vi "tagbit.vi"(9 "tag":string="A_B_C_D") -> (3 "tag cell":string[](array[string]))   [LabVIEW 2011]
uses:
  <vilib>/regexp/Match Regular Expression.xnode
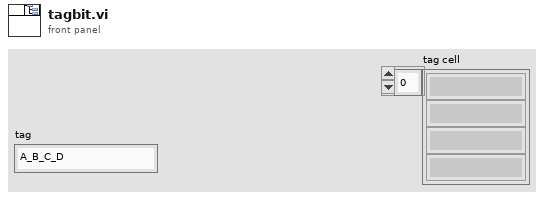
[diagram p1: front panel]
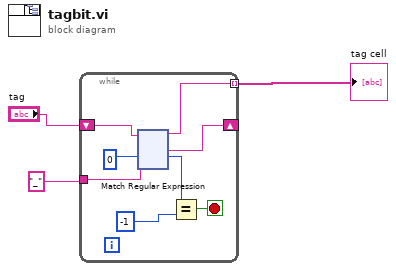
[diagram p0: block diagram]
diagram:
  n1 = while {
    tunnel: "_" ("regular expression") -> [w10]
    shift-right: [w4] -> _
    shift-left: "tag" -> [w11]
    tunnel: [w6] -> w1 mode=indexing
    stop <- w8 stop-if-true
    n2 = xnode "Match Regular Expression"("input string"=w11, "regular expression"=w10, "offset (0)"=0) -> ("before match"=w6:string, "after match"=w4:string, "offset past match"=w7:i32)  [unwired: 3 in, 2 out]
    n3 = Equal?(x=w7, y=-1) -> (x = y?=w8:bool)
  }
  "tag cell" <- w1
